vi "[P] Sin Wave 2.vi"   [LabVIEW 2014]
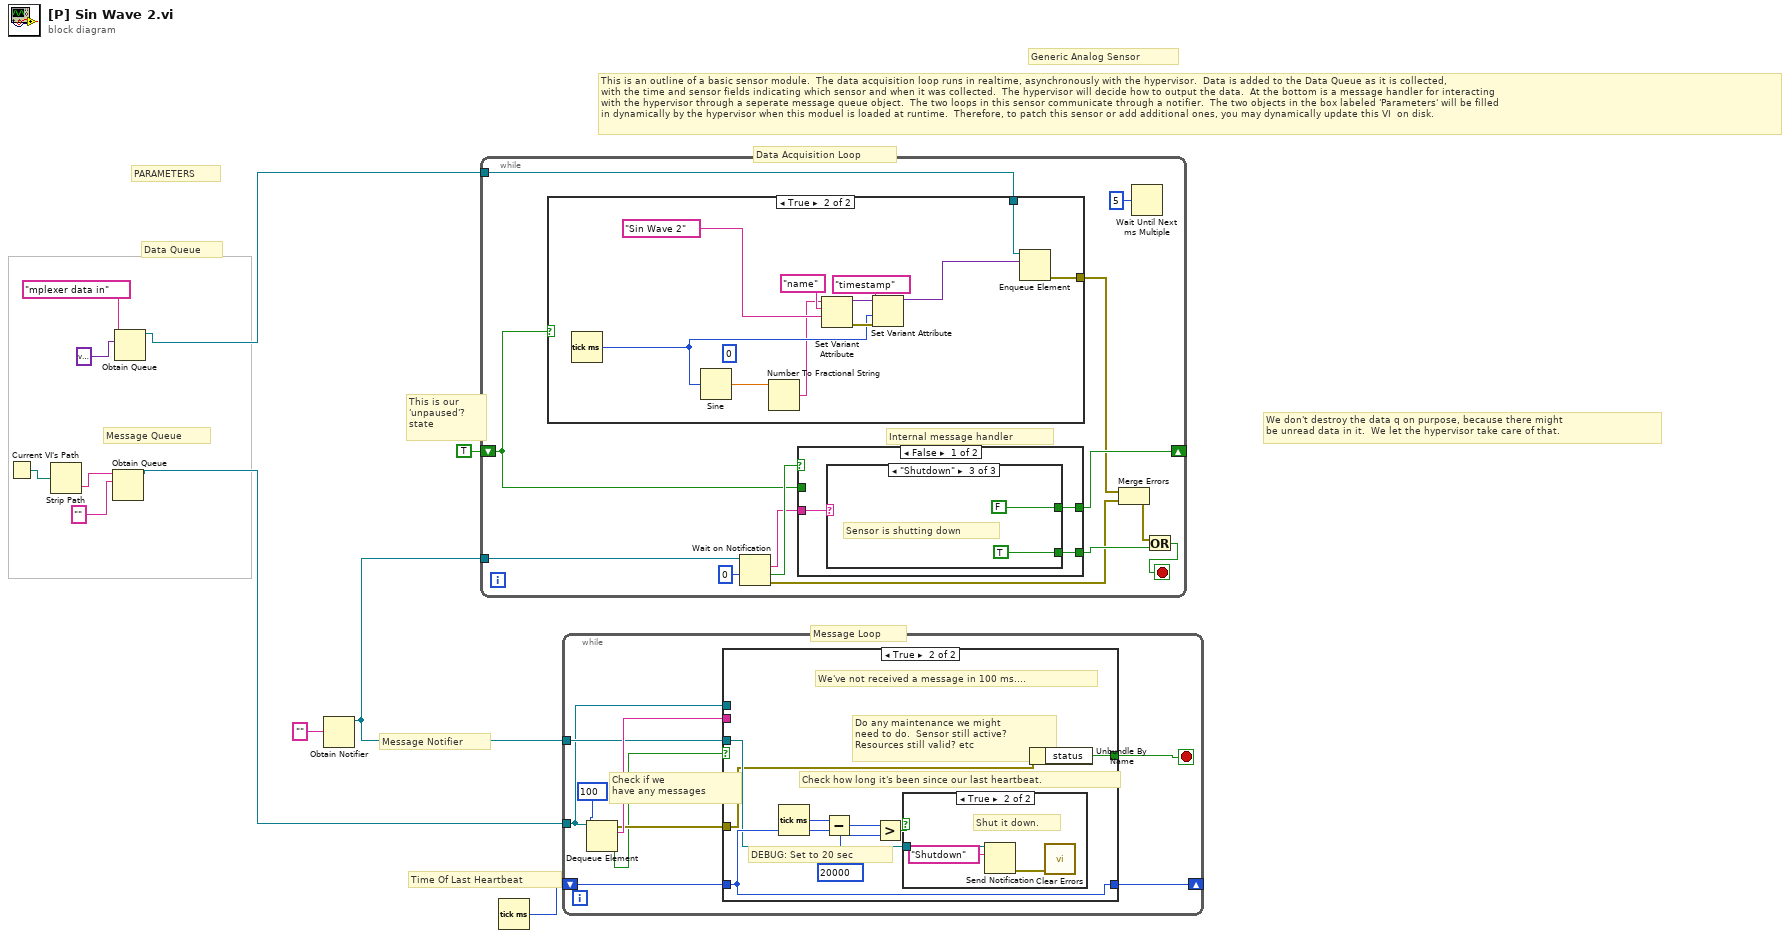
[diagram p0: block diagram]
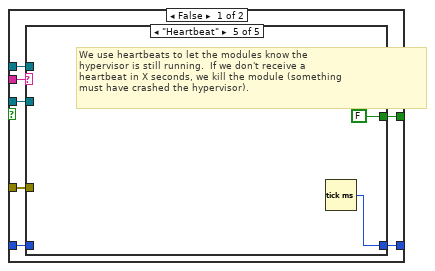
[diagram p2: hidden frame]
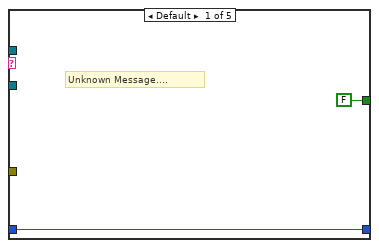
[diagram p3: hidden frame]
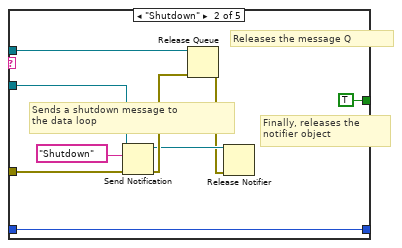
[diagram p4: hidden frame]
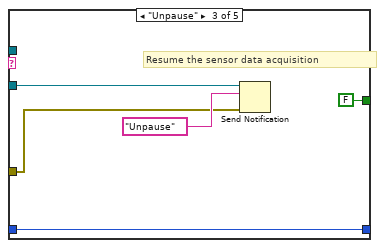
[diagram p5: hidden frame]
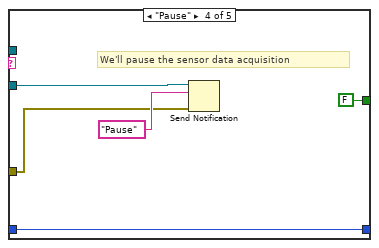
[diagram p6: hidden frame]
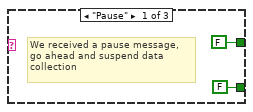
[diagram p9: hidden frame]
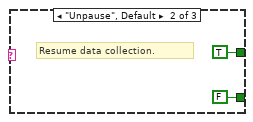
[diagram p10: hidden frame]
diagram:
  # "Time Of Last Heartbeat"
  # "This is an outline of a basic sensor module.  The data acquisition loop runs in realtime, asynchronously with the hypervisor.  Data is added to the Data Queue as it is collected,\nwith the time and sensor fields indicating which sensor and when it was collected.  The hypervisor will decide how to output the data.  At the bottom is a message handler for interacting\nwith the hypervisor through a seperate message queue object.  The two loops in this sensor communicate through a notifier.  The two objects in the box labeled 'Parameters' will be filled\nin dynamically by the hypervisor when this moduel is loaded at runtime.  Therefore, to patch this sensor or add additional ones, you may dynamically update this VI  on disk."
  # "This is our\n'unpaused'?\nstate"
  # "We don't destroy the data q on purpose, because there might\nbe unread data in it.  We let the hypervisor take care of that."
  # "Data Acquisition Loop"
  # "Message Loop"
  # "Message Notifier"
  # "Message Queue"
  # "Data Queue"
  # "PARAMETERS"
  # "Generic Analog Sensor"
  n1 = Current VI's Path() -> (path=w7:path)
  n2 = Strip Path(path=w7) -> (name=w6:string)  [unwired: 1 out]
  n3 = Obtain Queue(name (unnamed)=w6, element data type="") -> (queue out=w4:refnum<queue>)  [unwired: 3 in, 2 out]
  n4 = Obtain Queue(name (unnamed)="mplexer data in", element data type=variant) -> (queue out=w3:refnum<queue>)  [unwired: 3 in, 2 out]
  n5 = Obtain Notifier(notification data type="") -> (notifier out=w8:refnum<notifier>)  [unwired: 3 in, 2 out]
  n6 = while {
    tunnel: w3 -> [w16]
    tunnel: w8 -> [w24]
    shift-right: [w20] -> _
    shift-left: TRUE -> [w19]
    stop <- w15 stop-if-true
    # "Internal message handler"
    n7 = case shown="True" w19 {
      tunnel: w16 -> [_ w34]
      tunnel: [_ w33] -> w14
      frame False {
      }
      frame True {
        (unwired) u64 0 ("Fractional Time")
        n8 = Tick Count (ms)() -> (millisecond timer value=w27:u32)
        n9 = Sine(x=w27) -> (sin(x)=w35:dbl)
        n10 = Number To Fractional String(number=w35) -> (F-format string=w26:string)  [unwired: 3 in]
        n11 = Set Variant Attribute(Variant=w26, name="name", value="Sin Wave 2" ("Sensor Name")) -> (Variant out=w29:variant, error out=w30:errorcluster)  [unwired: 1 in, 1 out]
        n12 = Set Variant Attribute(Variant=w29, name="timestamp", value=w27, error in=w30) -> (Variant out=w25:variant)  [unwired: 2 out]
        n13 = Enqueue Element(queue=w34, element=w25) -> (error out=w33:errorcluster)  [unwired: 2 in, 2 out]
      }
    }
    n14 = Wait on Notification(notifier=w24, timeout in ms (-1)=0) -> (notification=w21:string, timed out?=w22:bool, error out=w13:errorcluster)  [unwired: 2 in, 1 out]
    n15 = case shown="False" w22 {
      tunnel: w21 -> [w38 _]
      tunnel: [w37 _] -> w18
      tunnel: [w36 w45] -> w20
      tunnel: w19 -> [_ w45]
      frame False {
        n16 = case shown="\"Shutdown\"" w38 {
          tunnel: [FALSE FALSE TRUE] -> w37
          tunnel: [FALSE TRUE FALSE] -> w36
          frame "Pause" {
            # "We received a pause message,\ngo ahead and suspend data collection"
          }
          frame "Unpause", Default {
            # "Resume data collection."
          }
          frame "Shutdown" {
            # "Sensor is shutting down"
          }
        }
      }
      frame True {
      }
    }
    n17 = Merge Errors(w14, w13) -> (w12:errorcluster)
    n18 = Wait Until Next ms Multiple(millisecond multiple=u32 5) -> ()  [unwired: 1 out]
    n19 = Or(x=w12, y=w18) -> (x .or. y?=w15:bool)
  }
  n20 = Tick Count (ms)() -> (millisecond timer value=w9:u32)
  n21 = while {
    tunnel: w4 -> [w51]
    tunnel: w8 -> [w52]
    shift-right: [w46] -> _
    shift-left: w9 -> [w47]
    stop <- w53 stop-if-true
    # "Check if we \nhave any messages"
    n22 = Dequeue Element(queue=w51, timeout in ms (-1)=100) -> (element=w54:string, timed out?=w48:bool, error out=w50:errorcluster)  [unwired: 1 in, 1 out]
    n23 = case shown="True" w48 {
      tunnel: w54 -> [w61 _]
      tunnel: [w60 w85] -> w53
      tunnel: w52 -> [w59 w87]
      tunnel: w51 -> [w58 _]
      tunnel: w50 -> [w57 w86]
      tunnel: w47 -> [w56 w88]
      tunnel: [w55 w88] -> w46
      frame False {
        n24 = case shown="\"Heartbeat\"" w61 {
          tunnel: [FALSE TRUE FALSE FALSE FALSE] -> w60
          tunnel: w59 -> [_ w70 w75 w79 _]
          tunnel: w58 -> [_ w71 _ _ _]
          tunnel: w57 -> [_ w69 w76 w80 _]
          tunnel: w56 -> [w62 w64 w73 w78 _]
          tunnel: [w62 w64 w73 w78 w84] -> w55
          frame Default {
            # "Unknown Message...."
          }
          frame "Shutdown" {
            # "Finally, releases the\nnotifier object"
            # "Releases the message Q"
            # "Sends a shutdown message to \nthe data loop"
            n25 = Send Notification(notification="Shutdown", notifier=w70, error in (no error)=w69) -> (notifier out=w66:refnum<notifier>, error out=w68:errorcluster)
            n26 = Release Queue(queue=w71, error in (no error)=w68) -> (error out=w65:errorcluster)  [unwired: 1 in, 2 out]
            n27 = Release Notifier(notifier=w66, error in (no error)=w65) -> ()  [unwired: 1 in, 3 out]
          }
          frame "Unpause" {
            # "Resume the sensor data acquisition"
            n28 = Send Notification(notification="Unpause", notifier=w75, error in (no error)=w76) -> ()  [unwired: 2 out]
          }
          frame "Pause" {
            # "We'll pause the sensor data acquisition"
            n29 = Send Notification(notification="Pause", notifier=w79, error in (no error)=w80) -> ()  [unwired: 2 out]
          }
          frame "Heartbeat" {
            # "We use heartbeats to let the modules know the \nhypervisor is still running.  If we don't receive a\nheartbeat in X seconds, we kill the module (something\nmust have crashed the hypervisor)."
            n30 = Tick Count (ms)() -> (millisecond timer value=w84:u32)
          }
        }
      }
      frame True {
        # "DEBUG: Set to 20 sec"
        # "Check how long it's been since our last heartbeat."
        # "Do any maintenance we might\nneed to do.  Sensor still active?\nResources still valid? etc"
        # "We've not received a message in 100 ms...."
        n31 = Tick Count (ms)() -> (millisecond timer value=w92:u32)
        n32 = Subtract(x=w92, y=w88) -> (x-y=w91:u32)
        n33 = Greater?(x=w91, y=u32 20000) -> (0:w89:bool)
        n34 = case shown="True" w89 {
          tunnel: w87 -> [_ w95]
          frame False {
          }
          frame True {
            # "Shut it down."
            n35 = Send Notification(notification="Shutdown", notifier=w95) -> (error out=w93:errorcluster)  [unwired: 1 in, 1 out]
            n36 = call <vilib>:"Clear Errors.vi"("error in (no error)"=w93) -> ()  [unwired: 5 in, 2 out]
          }
        }
        n37 = Unbundle By Name(w86) -> ("status"=w85:bool)
      }
    }
  }
